vi "Refprop tester.vi"(8 "error in (no error)":errorcluster) -> (0 "error out":errorcluster)   [LabVIEW 2015]
panel:
  out "REFPROP":bool
  out "REFPROP2":bool
  out "ALLPROPS0":bool
  out "ALLPROPS":bool
  out "ALLPROPS20":bool
  out "ALLPROPS1":bool
  out "REFPROP1":bool
  out "ABFLSH":bool
  out "GETENUM":bool
  out "FLAGS":bool
  out "ERRMSG":bool
  out "SETFLUIDS":bool
  out "SETPATH":bool
  out "SETMIXTURE":bool
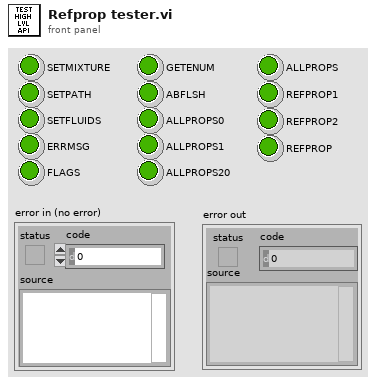
[diagram p1: front panel]
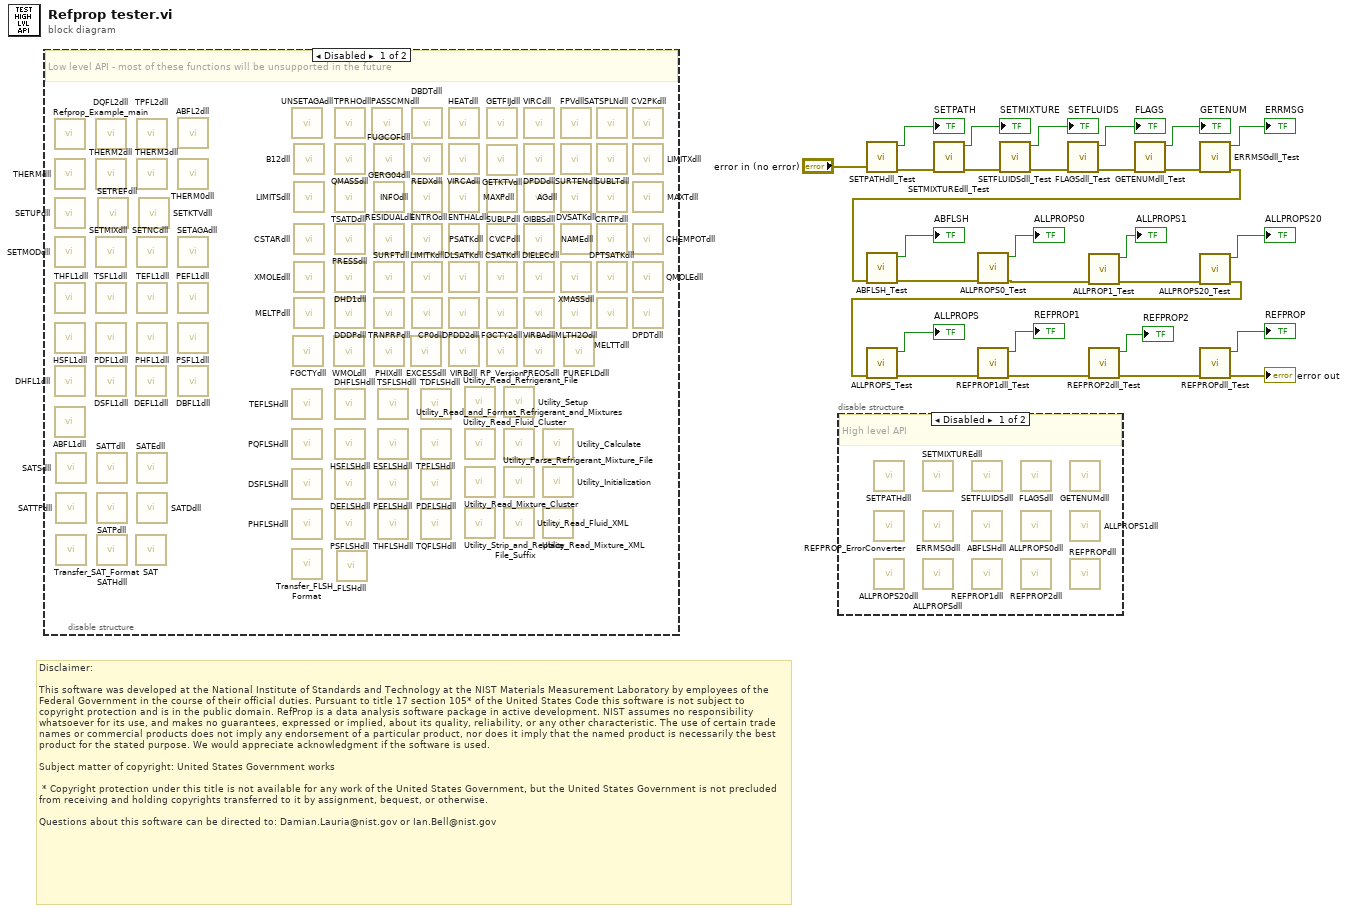
[diagram p0: block diagram]
diagram:
  # "Disclaimer:\n\nThis software was developed at the National Institute of Standards and Technology at the NIST Materials Measurement Laboratory by employees of the Federal Government in the course of their official duties. Pursuant to title 17 section 105* of the United States Code this software is not subject to copyright protection and is in the public domain. RefProp is a data analysis software package in active development. NIST assumes no responsibility whatsoever for its use, and makes no guarantees, expressed or implied, about its quality, reliability, or any other characteristic. The use of certain trade names or commercial products does not imply any endorsement of a particular product, nor does it imply that the named product is necessarily the best product for the stated purpose. We would appreciate acknowledgment if the software is used.\n \nSubject matter of copyright: United States Government works\n  \n * Copyright protection under this title is not available for any work of the United States Government, but the United States Government is not precluded from receiving and holding copyrights transferred to it by assignment, bequest, or otherwise.\n\nQuestions about this software can be directed to: Damian.Lauria@nist.gov or Ian.Bell@nist.gov"
  n1 = disable-structure shown="Disabled" {
    frame Disabled {
      # "Low level API - most of these functions will be unsupported in the future"
      n2 = call "Refprop_Example_main.vi"() -> ()  [unwired: 1 in]
      n3 = call "THERMdll.vi"() -> ()  [unwired: 10 in, 2 out]
      n4 = call "SETUPdll.vi"() -> ()  [unwired: 9 in, 3 out]
      n5 = call "SETMODdll.vi"() -> ()  [unwired: 10 in, 2 out]
      n6 = call "THFL1dll.vi"() -> ()  [unwired: 10 in, 2 out]
      n7 = call "HSFL1dll.vi"() -> ()  [unwired: 10 in, 2 out]
      n8 = call "DHFL1dll.vi"() -> ()  [unwired: 10 in, 2 out]
      n9 = call "ABFL1dll.vi"() -> ()  [unwired: 10 in, 2 out]
      n10 = call "SATSdll.vi"() -> ()  [unwired: 10 in, 2 out]
      n11 = call "SATTPdll.vi"() -> ()  [unwired: 10 in, 2 out]
      n12 = call "Transfer_SAT_Format.vi"() -> ()  [unwired: 11 in, 1 out]
      n13 = call "DQFL2dll.vi"() -> ()  [unwired: 10 in, 2 out]
      n14 = call "THERM2dll.vi"() -> ()  [unwired: 10 in, 2 out]
      n15 = call "SETMIXdll.vi"() -> ()  [unwired: 10 in, 2 out]
      n16 = call "TSFL1dll.vi"() -> ()  [unwired: 10 in, 2 out]
      n17 = call "PDFL1dll.vi"() -> ()  [unwired: 10 in, 2 out]
      n18 = call "DSFL1dll.vi"() -> ()  [unwired: 10 in, 2 out]
      n19 = call "SATTdll.vi"() -> ()  [unwired: 10 in, 2 out]
      n20 = call "SATPdll.vi"() -> ()  [unwired: 10 in, 2 out]
      n21 = call "SATHdll.vi"() -> ()  [unwired: 10 in, 2 out]
      n22 = call "SETREFdll.vi"() -> ()  [unwired: 10 in, 2 out]
      n23 = call "DEFL1dll.vi"() -> ()  [unwired: 10 in, 2 out]
      n24 = call-poly "SAT.vi"() -> ()  [unwired: 10 in, 2 out]
      n25 = call "TPFL2dll.vi"() -> ()  [unwired: 8 in, 4 out]
      n26 = call "THERM3dll.vi"() -> ()  [unwired: 10 in, 2 out]
      n27 = call "SETNCdll.vi"() -> ()  [unwired: 10 in, 2 out]
      n28 = call "TEFL1dll.vi"() -> ()  [unwired: 10 in, 2 out]
      n29 = call "PHFL1dll.vi"() -> ()  [unwired: 10 in, 2 out]
      n30 = call "SATEdll.vi"() -> ()  [unwired: 10 in, 2 out]
      n31 = call "SATDdll.vi"() -> ()  [unwired: 9 in, 3 out]
      n32 = call "SETKTVdll.vi"() -> ()  [unwired: 10 in, 2 out]
      n33 = call "ABFL2dll.vi"() -> ()  [unwired: 10 in, 2 out]
      n34 = call "THERM0dll.vi"() -> ()  [unwired: 10 in, 2 out]
      n35 = call "SETAGAdll.vi"() -> ()  [unwired: 9 in, 3 out]
      n36 = call "PEFL1dll.vi"() -> ()  [unwired: 10 in, 2 out]
      n37 = call "PSFL1dll.vi"() -> ()  [unwired: 10 in, 2 out]
      n38 = call "DBFL1dll.vi"() -> ()  [unwired: 10 in, 2 out]
      n39 = call "UNSETAGAdll.vi"() -> ()  [unwired: 11 in, 1 out]
      n40 = call "TEFLSHdll.vi"() -> ()  [unwired: 10 in, 2 out]
      n41 = call "PQFLSHdll.vi"() -> ()  [unwired: 10 in, 2 out]
      n42 = call "DSFLSHdll.vi"() -> ()  [unwired: 10 in, 2 out]
      n43 = call "PHFLSHdll.vi"() -> ()  [unwired: 10 in, 2 out]
      n44 = call "Transfer_FLSH_Format.vi"() -> ()  [unwired: 11 in, 1 out]
      n45 = call "FGCTYdll.vi"() -> ()  [unwired: 10 in, 2 out]
      n46 = call "B12dll.vi"() -> ()  [unwired: 10 in, 2 out]
      n47 = call "LIMITSdll.vi"() -> ()  [unwired: 10 in, 2 out]
      n48 = call "CSTARdll.vi"() -> ()  [unwired: 10 in, 2 out]
      n49 = call "XMOLEdll.vi"() -> ()  [unwired: 9 in, 3 out]
      n50 = call "MELTPdll.vi"() -> ()  [unwired: 10 in, 2 out]
      n51 = call "WMOLdll.vi"() -> ()  [unwired: 9 in, 3 out]
      n52 = call "TPRHOdll.vi"() -> ()  [unwired: 10 in, 2 out]
      n53 = call "QMASSdll.vi"() -> ()  [unwired: 10 in, 2 out]
      n54 = call "TSATDdll.vi"() -> ()  [unwired: 10 in, 2 out]
      n55 = call "PRESSdll.vi"() -> ()  [unwired: 10 in, 2 out]
      n56 = call "DHD1dll.vi"() -> ()  [unwired: 10 in, 2 out]
      n57 = call "DDDPdll.vi"() -> ()  [unwired: 10 in, 2 out]
      n58 = call "DHFLSHdll.vi"() -> ()  [unwired: 10 in, 2 out]
      n59 = call "HSFLSHdll.vi"() -> ()  [unwired: 10 in, 2 out]
      n60 = call "DEFLSHdll.vi"() -> ()  [unwired: 10 in, 2 out]
      n61 = call "PSFLSHdll.vi"() -> ()  [unwired: 10 in, 2 out]
      n62 = call-poly "FLSHdll.vi"() -> ()  [unwired: 10 in, 2 out]
      n63 = call "PASSCMNdll.vi"() -> ()  [unwired: 10 in, 2 out]
      n64 = call "FUGCOFdll.vi"() -> ()  [unwired: 10 in, 2 out]
      n65 = call "GERG04dll.vi"() -> ()  [unwired: 10 in, 2 out]
      n66 = call "RESIDUALdll.vi"() -> ()  [unwired: 10 in, 2 out]
      n67 = call "SURFTdll.vi"() -> ()  [unwired: 10 in, 2 out]
      n68 = call "TRNPRPdll.vi"() -> ()  [unwired: 10 in, 2 out]
      n69 = call "PHIXdll.vi"() -> ()  [unwired: 10 in, 2 out]
      n70 = call "TSFLSHdll.vi"() -> ()  [unwired: 10 in, 2 out]
      n71 = call "ESFLSHdll.vi"() -> ()  [unwired: 10 in, 2 out]
      n72 = call "PEFLSHdll.vi"() -> ()  [unwired: 10 in, 2 out]
      n73 = call "THFLSHdll.vi"() -> ()  [unwired: 10 in, 2 out]
      n74 = call "EXCESSdll.vi"() -> ()  [unwired: 10 in, 2 out]
      n75 = call "DBDTdll.vi"() -> ()  [unwired: 10 in, 2 out]
      n76 = call "REDXdll.vi"() -> ()  [unwired: 8 in, 4 out]
      n77 = call "INFOdll.vi"() -> ()  [unwired: 10 in, 2 out]
      n78 = call "ENTROdll.vi"() -> ()  [unwired: 10 in, 2 out]
      n79 = call "LIMITKdll.vi"() -> ()  [unwired: 10 in, 2 out]
      n80 = call "CP0dll.vi"() -> ()  [unwired: 8 in, 4 out]
      n81 = call "TDFLSHdll.vi"() -> ()  [unwired: 10 in, 2 out]
      n82 = call "TPFLSHdll.vi"() -> ()  [unwired: 10 in, 2 out]
      n83 = call "PDFLSHdll.vi"() -> ()  [unwired: 10 in, 2 out]
      n84 = call "TQFLSHdll.vi"() -> ()  [unwired: 10 in, 2 out]
      n85 = call "HEATdll.vi"() -> ()  [unwired: 10 in, 2 out]
      n86 = call "VIRCAdll.vi"() -> ()  [unwired: 10 in, 2 out]
      n87 = call "MAXPdll.vi"() -> ()  [unwired: 10 in, 2 out]
      n88 = call "ENTHALdll.vi"() -> ()  [unwired: 10 in, 2 out]
      n89 = call "DLSATKdll.vi"() -> ()  [unwired: 10 in, 2 out]
      n90 = call "DPDD2dll.vi"() -> ()  [unwired: 10 in, 2 out]
      n91 = call "VIRBdll.vi"() -> ()  [unwired: 10 in, 2 out]
      n92 = call "Utility_Read_Refrigerant_File.vi"() -> ()  [unwired: 8 in, 2 out]
      n93 = call "Utility_Read_Fluid_Cluster.vi"() -> ()  [unwired: 8 in, 2 out]
      n94 = call "Utility_Read_Mixture_Cluster.vi"() -> ()  [unwired: 8 in, 2 out]
      n95 = call "Utility_Strip_and_Replace_File_Suffix.vi"() -> ()  [unwired: 4 in, 2 out]
      n96 = call "GETFIJdll.vi"() -> ()  [unwired: 10 in, 2 out]
      n97 = call "GETKTVdll.vi"() -> ()  [unwired: 10 in, 2 out]
      n98 = call "SUBLPdll.vi"() -> ()  [unwired: 10 in, 2 out]
      n99 = call "PSATKdll.vi"() -> ()  [unwired: 10 in, 2 out]
      n100 = call "CSATKdll.vi"() -> ()  [unwired: 10 in, 2 out]
      n101 = call "FGCTY2dll.vi"() -> ()  [unwired: 10 in, 2 out]
      n102 = call "RP_Version.vi"() -> ()  [unwired: 10 in, 2 out]
      n103 = call "Utility_Setup.vi"() -> ()  [unwired: 7 in, 3 out]
      n104 = call "Utility_Read_and_Format_Refrigerant_and_Mixtures.vi"() -> ()  [unwired: 7 in, 3 out]
      n105 = call "Utility_Parse_Refrigerant_Mixture_File.vi"() -> ()  [unwired: 8 in, 2 out]
      n106 = call "Utility_Read_Fluid_XML.vi"() -> ()  [unwired: 11 in, 1 out]
      n107 = call "VIRCdll.vi"() -> ()  [unwired: 10 in, 2 out]
      n108 = call "DPDDdll.vi"() -> ()  [unwired: 10 in, 2 out]
      n109 = call "GIBBSdll.vi"() -> ()  [unwired: 9 in, 3 out]
      n110 = call "CVCPdll.vi"() -> ()  [unwired: 9 in, 3 out]
      n111 = call "DIELECdll.vi"() -> ()  [unwired: 10 in, 2 out]
      n112 = call "VIRBAdll.vi"() -> ()  [unwired: 10 in, 2 out]
      n113 = call "PREOSdll.vi"() -> ()  [unwired: 11 in, 1 out]
      n114 = call "Utility_Calculate.vi"() -> ()  [unwired: 9 in, 3 out]
      n115 = call "Utility_Initialization.vi"() -> ()  [unwired: 9 in, 3 out]
      n116 = call "Utility_Read_Mixture_XML.vi"() -> ()  [unwired: 11 in, 1 out]
      n117 = call "FPVdll.vi"() -> ()  [unwired: 10 in, 2 out]
      n118 = call "SURTENdll.vi"() -> ()  [unwired: 10 in, 2 out]
      n119 = call "AGdll.vi"() -> ()  [unwired: 10 in, 2 out]
      n120 = call "DVSATKdll.vi"() -> ()  [unwired: 10 in, 2 out]
      n121 = call "XMASSdll.vi"() -> ()  [unwired: 9 in, 3 out]
      n122 = call "MLTH2Odll.vi"() -> ()  [unwired: 8 in, 4 out]
      n123 = call "PUREFLDdll.vi"() -> ()  [unwired: 10 in, 2 out]
      n124 = call "SATSPLNdll.vi"() -> ()  [unwired: 8 in, 4 out]
      n125 = call "SUBLTdll.vi"() -> ()  [unwired: 10 in, 2 out]
      n126 = call "CRITPdll.vi"() -> ()  [unwired: 10 in, 2 out]
      n127 = call "NAMEdll.vi"() -> ()  [unwired: 10 in, 2 out]
      n128 = call "DPTSATKdll.vi"() -> ()  [unwired: 10 in, 2 out]
      n129 = call "MELTTdll.vi"() -> ()  [unwired: 10 in, 2 out]
      n130 = call "CV2PKdll.vi"() -> ()  [unwired: 10 in, 2 out]
      n131 = call "LIMITXdll.vi"() -> ()  [unwired: 10 in, 2 out]
      n132 = call "MAXTdll.vi"() -> ()  [unwired: 10 in, 2 out]
      n133 = call "CHEMPOTdll.vi"() -> ()  [unwired: 10 in, 2 out]
      n134 = call "QMOLEdll.vi"() -> ()  [unwired: 10 in, 2 out]
      n135 = call "DPDTdll.vi"() -> ()  [unwired: 10 in, 2 out]
    }
    frame Enabled {
    }
  }
  n136 = disable-structure shown="Disabled" {
    frame Disabled {
      # "High level API"
      n137 = call "SETPATHdll.vi"() -> ()  [unwired: 9 in, 3 out]
      n138 = call "REFPROP_ErrorConverter.vi"() -> ()  [unwired: 11 in, 1 out]
      n139 = call "ALLPROPS20dll.vi"() -> ()  [unwired: 10 in, 2 out]
      n140 = call "SETMIXTUREdll.vi"() -> ()  [unwired: 8 in, 4 out]
      n141 = call "ERRMSGdll.vi"() -> ()  [unwired: 8 in, 4 out]
      n142 = call "ALLPROPSdll.vi"() -> ()  [unwired: 10 in, 2 out]
      n143 = call "SETFLUIDSdll.vi"() -> ()  [unwired: 8 in, 4 out]
      n144 = call "ABFLSHdll.vi"() -> ()  [unwired: 10 in, 2 out]
      n145 = call "REFPROP1dll.vi"() -> ()  [unwired: 10 in, 2 out]
      n146 = call "FLAGSdll.vi"() -> ()  [unwired: 10 in, 2 out]
      n147 = call "ALLPROPS0dll.vi"() -> ()  [unwired: 10 in, 2 out]
      n148 = call "REFPROP2dll.vi"() -> ()  [unwired: 10 in, 2 out]
      n149 = call "GETENUMdll.vi"() -> ()  [unwired: 10 in, 2 out]
      n150 = call "ALLPROPS1dll.vi"() -> ()  [unwired: 10 in, 2 out]
      n151 = call "REFPROPdll.vi"() -> ()  [unwired: 10 in, 2 out]
    }
    frame Enabled {
    }
  }
  n152 = call "SETPATHdll_Test.vi"("error in (no error)"="error in (no error)") -> ("error out"=w29:errorcluster, "Passed?"=→"SETPATH":bool)  [unwired: 9 in]
  n153 = call "SETMIXTUREdll_Test.vi"("error in (no error)"=w29) -> ("error out"=w28:errorcluster, "Passed?"=→"SETMIXTURE":bool)  [unwired: 9 in]
  n154 = call "SETFLUIDSdll_Test.vi"("error in (no error)"=w28) -> ("error out"=w27:errorcluster, "Passed?"=→"SETFLUIDS":bool)  [unwired: 9 in]
  n155 = call "FLAGSdll_Test.vi"("error in (no error)"=w27) -> ("error out"=w26:errorcluster, "Passed?"=→"FLAGS":bool)  [unwired: 9 in]
  n156 = call "GETENUMdll_Test.vi"("error in (no error)"=w26) -> ("error out"=w25:errorcluster, "Passed?"=→"GETENUM":bool)  [unwired: 9 in]
  n157 = call "ERRMSGdll_Test.vi"("error in (no error)"=w25) -> ("error out"=w17:errorcluster, "Passed?"=→"ERRMSG":bool)  [unwired: 9 in]
  n158 = call "ABFLSH_Test.vi"("error in (no error)"=w17) -> ("error out"=w8:errorcluster, "Passed?"=→"ABFLSH":bool)  [unwired: 9 in]
  n159 = call "ALLPROPS0_Test.vi"("error in (no error)"=w8) -> ("error out"=w7:errorcluster, "Passed?"=→"ALLPROPS0":bool)  [unwired: 9 in]
  n160 = call "ALLPROP1_Test.vi"("error in (no error)"=w7) -> ("error out"=w13:errorcluster, "Passed?"=→"ALLPROPS1":bool)  [unwired: 9 in]
  n161 = call "ALLPROPS20_Test.vi"("error in (no error)"=w13) -> ("error out 2"=w12:errorcluster, "Passed?"=→"ALLPROPS20":bool)  [unwired: 9 in]
  n162 = call "ALLPROPS_Test.vi"("error in (no error)"=w12) -> ("error out"=w10:errorcluster, "Passed?"=→"ALLPROPS":bool)  [unwired: 9 in]
  n163 = call "REFPROP1dll_Test.vi"("error in (no error)"=w10) -> ("error out"=w5:errorcluster, "Passed?"=→"REFPROP1":bool)  [unwired: 9 in]
  n164 = call "REFPROP2dll_Test.vi"("error in (no error)"=w5) -> ("error out"=w3:errorcluster, "Passed?"=→"REFPROP2":bool)  [unwired: 9 in]
  n165 = call "REFPROPdll_Test.vi"("error in (no error)"=w3) -> ("error out"=→"error out":errorcluster, "Passed?"=→"REFPROP":bool)  [unwired: 9 in]
